vi "Create SBlock.vi"   [LabVIEW 2020, in "CIRCUS_uServices.lvlib" / "Run Utilities.lvlib" / "Schedule Block.lvclass"]
uses:
  Schedule Block.lvclass
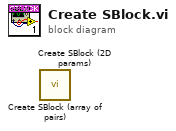
[diagram p0: block diagram]
diagram:
  n1 = call "Create SBlock (array of pairs).vi"() -> ()  [unwired: 13 in, 3 out]
  n2 = call "Create SBlock (2D params).vi"() -> ()  [unwired: 13 in, 3 out]
